vi "2. Enable and Disable Time References.vi"() -> ()   [LabVIEW 2019]
doc: "Demonstrates how to monitor and configure IEEE 1588-2008 and IEEE 802.1AS-2011 time references running on a real-time system."
uses:
  <instrlib>/niSync/niSync.llb/niSync Initialize (Default).vi
panel:
  in  "Persist?":bool
  out "error out":errorcluster
  out "TR to Toggle":string caption="Time Reference to Toggle Enable/Disable State"
  in  "Toggle Enable/Disable Button":bool
  in  "Cancel Button":bool
  in  "Multicolumn Listbox":i32(listbox)=-1
  in  "NI-Sync Resource":tag
  # "- Select a NI-Sync Resource to query for enabled and disabled time references.\n- Select a time reference in the listbox to toggle its enabled state. Confirm the time reference name in the \"Time Reference to Enable/Disable State\" label.\n- Select the \"Persist?\" toggle if the new enabled state should persist across device reboots. Leave unselected if rebooting should revert the change.\n- Click \"Toggle Enable/Disable State\" to change the enabled state, \"Cancel\" to quit without making any changes."
  # "Overview: Demonstrates how to monitor and configure IEEE 1588-2008 and IEEE 802.1AS-2011 time references running on a real-time system.\nRequirements: Runs on Windows and LinuxRT hosts to configure and monitor LinuxRT devices.\nInstructions:\n1. Select the resource to monitor/configure in the NI-Sync Resource dropdown.\n2. Use the tabs to switch to the protcol of interest.\n3. Monitor the enabled time references of this type in the table.\n4. To configure properties of a time reference:\n     a) Select the 1588 Time Reference to Configure.\n     b) Set properties to desired values.\n     c) Enable the Persist? Boolean if you would like these settings to persist across reboots.\n     d) Select Apply to commit the desired settings."
  # "* NOTE: Time references typically cannot share network interfaces, and therefore should not be enabled if another enabled time reference is using the same interface. In order to change time references on an interface, first disable any other time references using that interface, then enable the desired time reference."
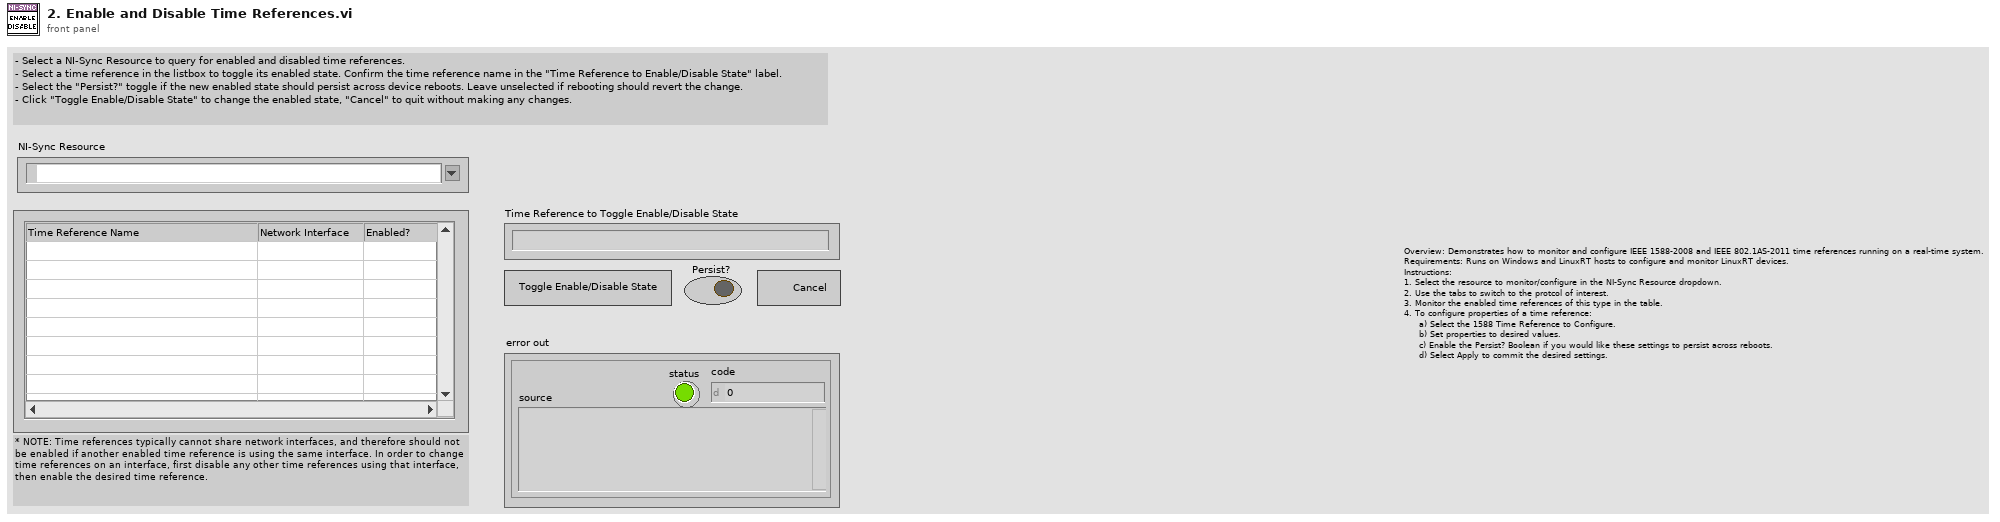
[diagram p1: front panel]
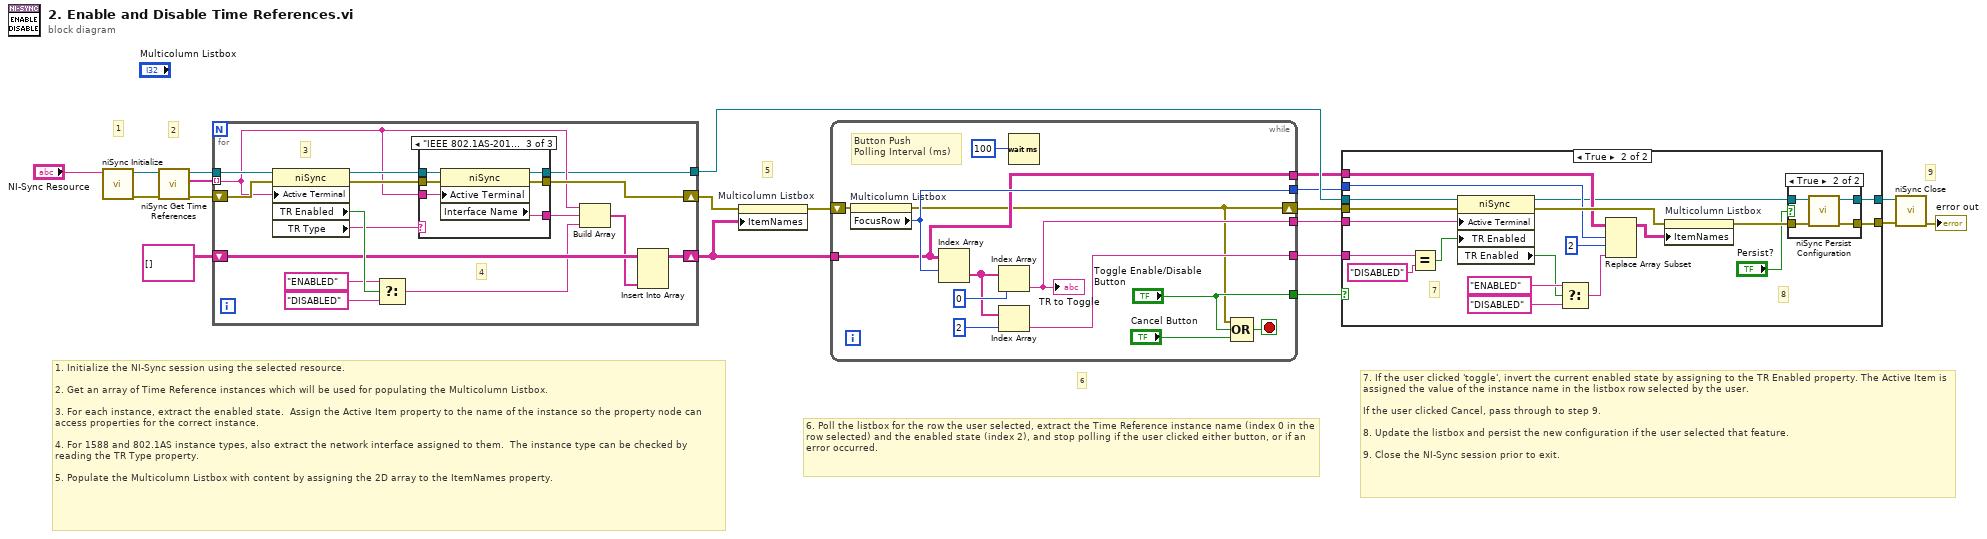
[diagram p0: block diagram]
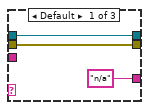
[diagram p4: hidden frame]
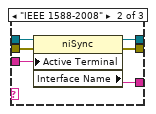
[diagram p5: hidden frame]
diagram:
  # "6"
  # "9"
  # "5"
  # "7. If the user clicked 'toggle', invert the current enabled state by assigning to the TR Enabled property. The Active Item is assigned the value of the instance name in the listbox row selected by the user.\n\nIf the user clicked Cancel, pass through to step 9.\n\n8. Update the listbox and persist the new configuration if the user selected that feature.\n\n9. Close the NI-Sync session prior to exit."
  # "6. Poll the listbox for the row the user selected, extract the Time Reference instance name (index 0 in the row selected) and the enabled state (index 2), and stop polling if the user clicked either button, or if an error occurred."
  # "2"
  # "1"
  # "1. Initialize the NI-Sync session using the selected resource.\n\n2. Get an array of Time Reference instances which will be used for populating the Multicolumn Listbox.\n\n3. For each instance, extract the enabled state.  Assign the Active Item property to the name of the instance so the property node can access properties for the correct instance.\n\n4. For 1588 and 802.1AS instance types, also extract the network interface assigned to them.  The instance type can be checked by reading the TR Type property.\n\n5. Populate the Multicolumn Listbox with content by assigning the 2D array to the ItemNames property."
  n1 = call-poly <instrlib>:"niSync Initialize.vi"("resource name"="NI-Sync Resource") -> ("error out"=w19:errorcluster, "instrument handle out"=w18:refnum<k15>)  [unwired: 9 in]
  n2 = call <instrlib>:"niSync Get Time References.vi"("error in (no error)"=w19, "instrument handle"=w18) -> ("error out"=w13:errorcluster, "time references"=w16:string[], "instrument handle out"=w17:refnum<k15>)  [unwired: 7 in]
  n3 = for {
    tunnel: w17 -> [w36]
    tunnel: w16 -> [w22] mode=indexing
    shift-right: [w32] -> w3
    shift-left: string[][] [] ("Item Names") -> [w31]
    shift-right: [w23] -> w14
    shift-left: w13 -> [w29]
    tunnel: [w21] -> w8
    # "4"
    # "3"
    n4 = property class="niSync"(reference=w36, error in=w29, "Active Terminal"=w22) -> (reference out=w25:refnum<k15>, error out=w26:errorcluster, "TR Enabled"=w35:bool, "TR Type"=w27:string)
    n5 = Select(t="ENABLED", s=w35, f="DISABLED") -> (s? t:f=w28:string)
    n6 = case shown="\"IEEE 802.1AS-2011\"" w27 {
      tunnel: w26 -> [w38 w45 w51]
      tunnel: w25 -> [w37 w44 w50]
      tunnel: ["n/a" ("Interface Name") w42 w48] -> w24
      tunnel: [w38 w43 w49] -> w23
      tunnel: w22 -> [_ w41 w47]
      tunnel: [w37 w40 w46] -> w21
      frame Default {
      }
      frame "IEEE 1588-2008" {
        n7 = property class="niSync"(reference=w44, error in=w45, "Active Terminal"=w41) -> (reference out=w40:refnum<k15>, error out=w43:errorcluster, "Interface Name"=w42:string)
      }
      frame "IEEE 802.1AS-2011" {
        n8 = property class="niSync"(reference=w50, error in=w51, "Active Terminal"=w47) -> (reference out=w46:refnum<k15>, error out=w49:errorcluster, "Interface Name"=w48:string)
      }
    }
    n9 = Build Array(w22, w24, w28) -> (w30:string[])
    n10 = Insert Into Array(array=w31, new element=w30) -> (w32:string[][])  [unwired: 2 in]
  }
  n11 = property on="Multicolumn Listbox" class="MCListbox (strict)"(error in=w14, "ItemNames"=w3) -> (error out=w4:errorcluster)  [unwired: 1 in, 1 out]
  n12 = while {
    shift-right: [w53] -> w7
    shift-left: w4 -> [w63]
    tunnel: [w62] -> w6
    tunnel: ["Toggle Enable/Disable Button"] -> w12
    tunnel: [w57] -> w9
    tunnel: [w56] -> w2
    tunnel: [w54] -> w1
    tunnel: w3 -> [w54]
    stop <- w61 stop-if-true
    # "Button Push\nPolling Interval (ms)"
    n13 = property on="Multicolumn Listbox" class="MCListbox (strict)"(error in=w63) -> (error out=w53:errorcluster, "FocusRow"=w56:i32)  [unwired: 1 in, 1 out]
    n14 = Index Array(array=w54, index (row)=w56) -> (element=w58:string[])  [unwired: 1 in]
    n15 = Index Array(array=w58, index=0) -> (element=w62:string)
    "TR to Toggle" <- w62
    n16 = Index Array(array=w58, index=2) -> (element=w57:string)
    n17 = Wait (ms)(milliseconds to wait=u32 100) -> ()  [unwired: 1 out]
    n18 = Compound Arithmetic op=OR(w53, "Toggle Enable/Disable Button", "Cancel Button") -> (w61:bool)
  }
  n19 = case shown="True" w12 {
    tunnel: w8 -> [w66 w81]
    tunnel: w7 -> [w65 w82]
    tunnel: [w66 w68] -> w11
    tunnel: [w65 w67] -> w10
    tunnel: w6 -> [_ w83]
    tunnel: w9 -> [_ w86]
    tunnel: w2 -> [_ w74]
    tunnel: w1 -> [_ w73]
    frame False {
    }
    frame True {
      # "7"
      # "8"
      n20 = Equal?(x=w86, y="DISABLED") -> (x = y?=w84:bool)
      n21 = property class="niSync"(reference=w81, error in=w82, "Active Terminal"=w83, "TR Enabled"=w84) -> (reference out=w70:refnum<k15>, error out=w79:errorcluster, "TR Enabled"=w75:bool)
      n22 = Select(t="ENABLED", s=w75, f="DISABLED") -> (s? t:f=w76:string)
      n23 = Replace Array Subset(array=w73, new element=w76, index (row)=w74, index (col)=2 ("disabled index (col)")) -> (w72:string[][])
      n24 = property on="Multicolumn Listbox" class="MCListbox (strict)"(error in=w79, "ItemNames"=w72) -> (error out=w71:errorcluster)  [unwired: 1 in, 1 out]
      n25 = case shown="True" "Persist?" {
        tunnel: w71 -> [w87 w92]
        tunnel: w70 -> [w88 w91]
        tunnel: [w88 w90] -> w68
        tunnel: [w87 w89] -> w67
        frame False {
        }
        frame True {
          n26 = call <instrlib>:"niSync Persist Configuration.vi"("error in (no error)"=w92, "instrument handle"=w91) -> ("error out"=w89:errorcluster, "instrument handle out"=w90:refnum<k15>)  [unwired: 8 in]
        }
      }
    }
  }
  n27 = call <instrlib>:"niSync Close.vi"("error in (no error)"=w10, "instrument handle"=w11) -> ("error out"=→"error out":errorcluster)  [unwired: 9 in]
